vi "Sort and Index (I32).vi"(4 "X":i32[](array[numeric]), 5 "Descending":bool) -> (0 "Index":i32[](array[numeric]), 1 "Sort(X)":i32[](array[numeric]))   [LabVIEW 2020]
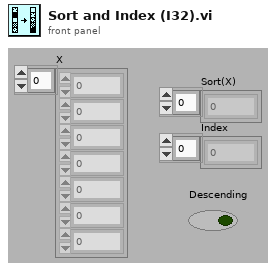
[diagram p1: front panel]
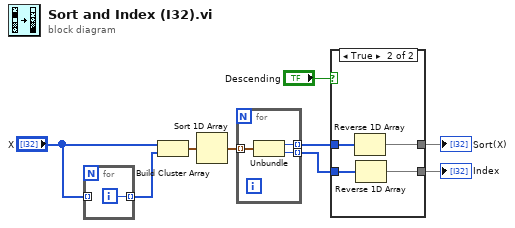
[diagram p0: block diagram]
diagram:
  n1 = for {
    tunnel: "X" -> [_] mode=indexing
    tunnel: [w10] -> w6 mode=indexing
    i -> [w10]
  }
  n2 = Build Cluster Array("X", w6) -> (w9:cluster{"value":i32, i32}[])
  n3 = Sort 1D Array(array=w9) -> (sorted array=w8:cluster{"value":i32, i32}[])
  n4 = for {
    tunnel: w8 -> [w13] mode=indexing
    tunnel: [w12] -> w2 mode=indexing
    tunnel: [w11] -> w4 mode=indexing
    n5 = Unbundle(w13) -> ("value"=w11:i32, w12:i32)
  }
  n6 = case shown="True" "Descending" {
    tunnel: w4 -> [w15 w19]
    tunnel: [w15 w18] -> w3
    tunnel: w2 -> [w14 w17]
    tunnel: [w14 w16] -> w1
    frame False {
    }
    frame True {
      n7 = Reverse 1D Array(array=w19) -> (reversed array=w18:i32[])
      n8 = Reverse 1D Array(array=w17) -> (reversed array=w16:i32[])
    }
  }
  "Sort(X)" <- w3
  "Index" <- w1
